vi "Visualise.vi"(10 "Rope in":cluster{"x":i64, "y":i64}[](array[cluster]), 11 "XYGraph in":refnum<vi>) -> (2 "Rope out":cluster{"x":i64, "y":i64}[](array[cluster]), 3 "XY Graph out":refnum<vi>)   [LabVIEW 2021, in "d9.lvlib"]
uses:
  d9.lvlib
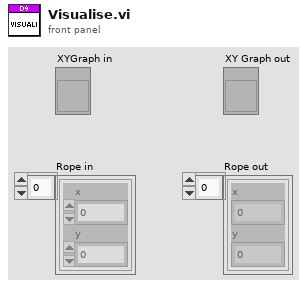
[diagram p1: front panel]
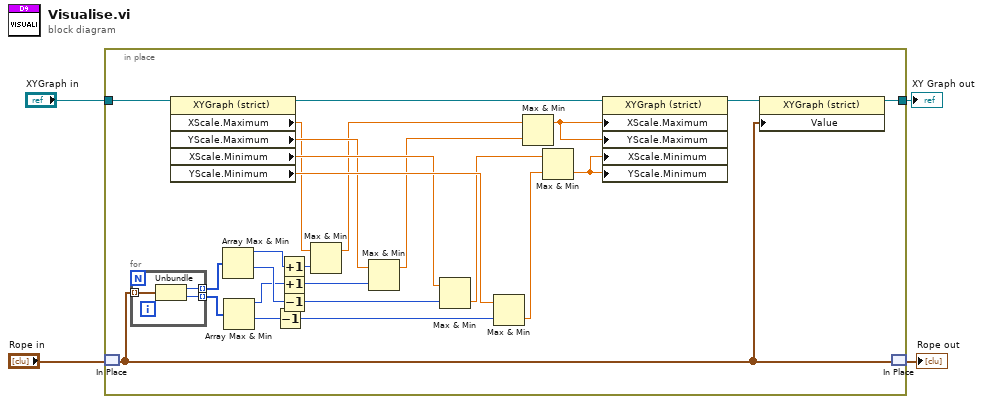
[diagram p0: block diagram]
diagram:
  n1 = in-place {
    in-place-border: "XYGraph in" -> [w27]
    in-place-border: [w19] -> w3
    n2 = in-place-match #1("Rope in") -> (w11:cluster{"x":i64, "y":i64}[])
    n3 = for {
      tunnel: w11 -> [w32] mode=indexing
      tunnel: [w31] -> w10 mode=indexing
      tunnel: [w30] -> w7 mode=indexing
      n4 = Unbundle(w32) -> ("x"=w31:i64, "y"=w30:i64)
    }
    n5 = property on="Property Node" class="XYGraph (strict)"(reference=w27) -> (reference out=w28:refnum<vi>, "XScale.Maximum"=w20:dbl, "YScale.Maximum"=w23:dbl, "XScale.Minimum"=w25:dbl, "YScale.Minimum"=w26:dbl)  [unwired: 1 in, 1 out]
    n6 = Array Max & Min(array=w10) -> (max value=w9:i64, min value=w8:i64)  [unwired: 2 out]
    n7 = Array Max & Min(array=w7) -> (max value=w6:i64, min value=w5:i64)  [unwired: 2 out]
    n8 = Decrement(x=w5) -> (x-1=w12:i64)
    n9 = Increment(x=w9) -> (x+1=w21:i64)
    n10 = Increment(x=w6) -> (x+1=w22:i64)
    n11 = Decrement(x=w8) -> (x-1=w24:i64)
    n12 = Max & Min(x=w20, y=w21) -> (max(x,y)=w17:dbl)  [unwired: 1 out]
    n13 = Max & Min(x=w23, y=w22) -> (max(x,y)=w18:dbl)  [unwired: 1 out]
    n14 = Max & Min(x=w25, y=w24) -> (min(x,y)=w15:dbl)  [unwired: 1 out]
    n15 = Max & Min(x=w26, y=w12) -> (min(x,y)=w14:dbl)  [unwired: 1 out]
    n16 = Max & Min(x=w17, y=w18) -> (max(x,y)=w16:dbl)  [unwired: 1 out]
    n17 = Max & Min(x=w15, y=w14) -> (min(x,y)=w13:dbl)  [unwired: 1 out]
    n18 = property on="Property Node" class="XYGraph (strict)"(reference=w28, "XScale.Maximum"=w16, "YScale.Maximum"=w16, "XScale.Minimum"=w13, "YScale.Minimum"=w13) -> (reference out=w29:refnum<vi>)  [unwired: 1 in, 1 out]
    n19 = property class="XYGraph (strict)"(reference=w29, "Value"=w11) -> (reference out=w19:refnum<vi>)  [unwired: 1 in, 1 out]
    n20 = in-place-match #1(w11) -> (→"Rope out":cluster{"x":i64, "y":i64}[])
  }
  "XY Graph out" <- w3
